vi "Serial write and read v0.2.vi"(1 "Termination char\n(0xA = '\\n' = LF)\n(0xD = '\\r' = CR)":u8=10 format="%.0x", 2 "Enable Termination\nChar (T)":bool=TRUE, 3 "parity":u16(ring) items=["None", "Odd", "Even", "Mark", "Space"], 4 "stop bits":u16(ring)=10 items=["1.0"=10, "1.5"=15, "2.0"=20], 5 "string to write":string="ZR", 6 "flow control":u16(ring) items=["None"=0, "XON/XOFF"=1, "RTS/CTS"=2, "DTR/DSR"=4], 7 "bytes to read":u32=5, 8 "Serial Settings:Serial End Mode for Reads":u16(ring)=2 items=["None", "LastBit", "TermChar"], 9 "Timeout (ms)":u32=10000, 11 "error in (no error)":errorcluster, 12 "VISA resource name":refnum<visa-resource-name>="COM8", 13 "baud rate":u32=9600, 14 "data bits":u16=8 min=5 max=8 step=1) -> (10 "read string":string, 15 "error out":errorcluster)   [LabVIEW 2016]
doc: "The Basic Serial Read and Write example performs a Serial Port Read, a Serial Port Write, or a combination of these actions. The user selects the actions (read or write) on the front panel. If both are selected, the VI will write the data first, read data, and then close the VISA session that is opened to the port. This VI will wait until the specified number of bytes is received at the port. Only the number of bytes specified will be read.\n\nINSTRUCTIONS:\n1) Select the serial resource and configuration parameters (baud rate, data bits, parity, stop bits, flow control).\n2) Select the operations to be performed. \n3) Connect the serial port to your device. If no device is available, perform a loopback test by doing one of the following. Short pins 2 and 3 on a RS-232 cable or short pin 4 to pin 8 and pin 5 to pin 9 on a RS-485/422 cable. \n4) Run the VI to see the data read. (The \"read string\" will match the \"string to write\" if a loopback test was performed.)\n\nNote: The parameters set for the serial port must match the parameters of the connected instrument or device. In this example, the bytes to read parameter specifies the number of bytes that the serial port reads. If there were more bytes at the port than the number specified in bytes to read, those bytes would not be read. Also, if you specify to read more bytes than the number of bytes actually read, you might receive a timeout error message.\n\nOn the block diagram, the Configure Serial Port VI sets the configuration parameters. The front panel displays the controls used to configure the basic parameters, such as baud rate, data bits, and parity. Constants configure the other parameters the user probably does not need set. After the VISA Configure Serial Port VI opens the VISA session and configures the port, the VI passes the VISA resource name to other VIs that perform operations on that VISA resource. The VISA Write function sends a command to the serial device and the VISA Read function returns data based on the command. The VISA Close function then closes the reference to the serial device. It is important to close the reference; otherwise communication through with that port through protocols other than VISA might not be possible."
panel:
  # "Select the serial resource and the operations (Read, Write, or both) to be performed.  If both are selected, the VI will write the data first, read data and then close the VISA session that is opened to the port.  This VI will wait until the specified number of bytes is received at the port. Only the number of bytes specified will be read."
  # "For additional information select File >> VI Properties >> Documentation"
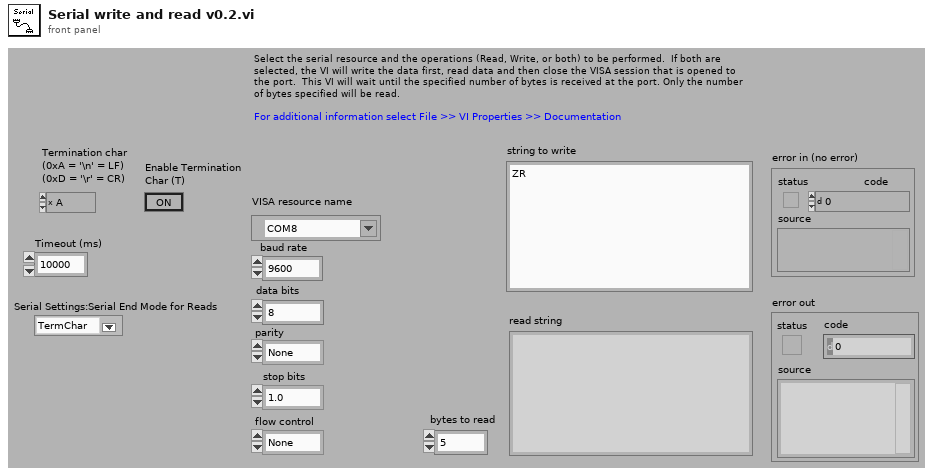
[diagram p1: front panel]
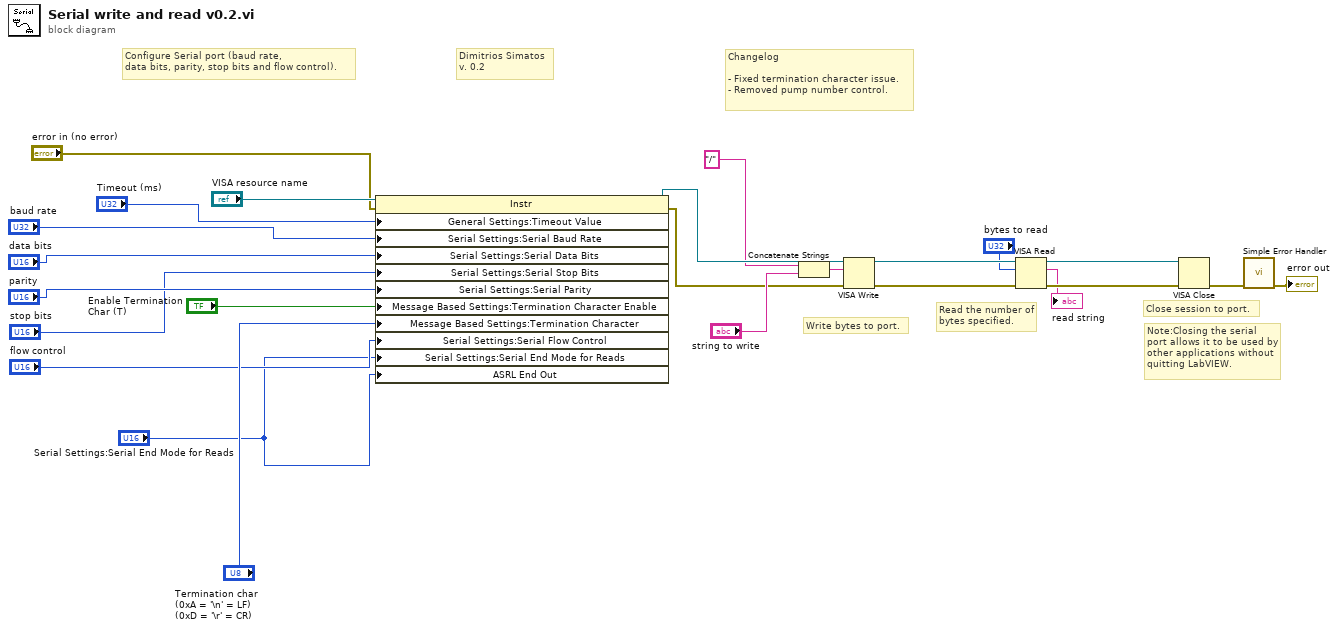
[diagram p0: block diagram]
diagram:
  # "Dimitrios Simatos\nv. 0.2"
  # "Changelog\n\n- Fixed termination character issue.\n- Removed pump number control."
  # "Read the number of bytes specified."
  # "Write bytes to port."
  # "Note:Closing the serial port allows it to be used by other applications without\nquitting LabVIEW."
  # "Configure Serial port (baud rate,\ndata bits, parity, stop bits and flow control)."
  # "Close session to port."
  n1 = property class="Instr"(reference="VISA resource name", error in="error in (no error)", "General Settings:Timeout Value"="Timeout (ms)", "Serial Settings:Serial Baud Rate"="baud rate", "Serial Settings:Serial Data Bits"="data bits", "Serial Settings:Serial Stop Bits"="stop bits", "Serial Settings:Serial Parity"="parity", "Message Based Settings:Termination Character Enable"="Enable Termination\nChar (T)", "Message Based Settings:Termination Character"="Termination char\n(0xA = '\\n' = LF)\n(0xD = '\\r' = CR)", "Serial Settings:Serial Flow Control"="flow control", "Serial Settings:Serial End Mode for Reads"="Serial Settings:Serial End Mode for Reads", "ASRL End Out"="Serial Settings:Serial End Mode for Reads") -> (reference out=w6:refnum<visa-resource-name>, error out=w5:errorcluster)
  n2 = Concatenate Strings("/" ("Start command"), "string to write") -> (w4:string)
  n3 = VISA Write(VISA resource name=w6, write buffer=w4, error in (no error)=w5) -> (VISA resource name out=w20:refnum<visa-resource-name>, error out=w24:errorcluster)  [unwired: 1 out]
  n4 = VISA Read(VISA resource name=w20, byte count="bytes to read", error in (no error)=w24) -> (VISA resource name out=w22:refnum<visa-resource-name>, read buffer=→"read string":string, error out=w23:errorcluster)  [unwired: 1 out]
  n5 = VISA Close(VISA resource name=w22, error in (no error)=w23) -> (error out=w21:errorcluster)
  n6 = call <vilib>:"Simple Error Handler.vi"("error in (no error)"=w21) -> ("error out"=→"error out":errorcluster)  [unwired: 4 in, 4 out]
